vi "NewCore.vi"(8 "error in (no error)":errorcluster, 10 "ParamsArray":variant[](array[variant]), 11 "DoorNeedingSpell":refnum<class "DoorNeedingSpell.lvclass">) -> (0 "error out":errorcluster, 3 "DoorNeedingSpell":refnum<class "DoorNeedingSpell.lvclass">)   [LabVIEW 2020, in "DoorNeedingSpell.lvclass"]
uses:
  DoorNeedingSpell.lvclass
  Private/TypeDef/privateData.ctl
  DoorNeedingSpell.lvclass/DoorNeedingSpell.ctl
  Door/Door.lvclass
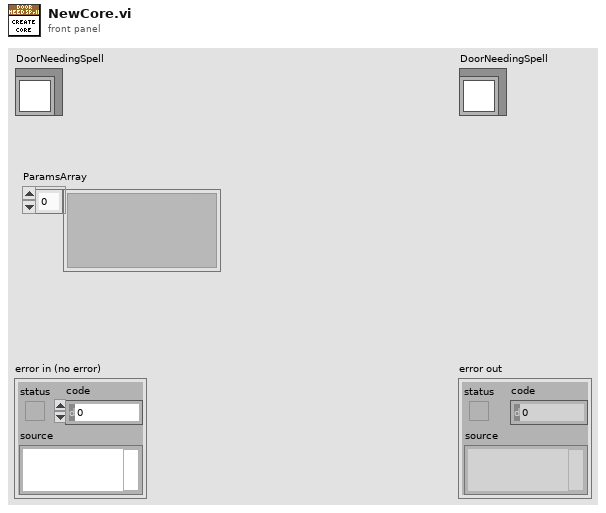
[diagram p1: front panel]
types:
  T1 = typedef "DoorNeedingSpell.lvclass/privateData.ctl" = cluster{"Dummy":i32}
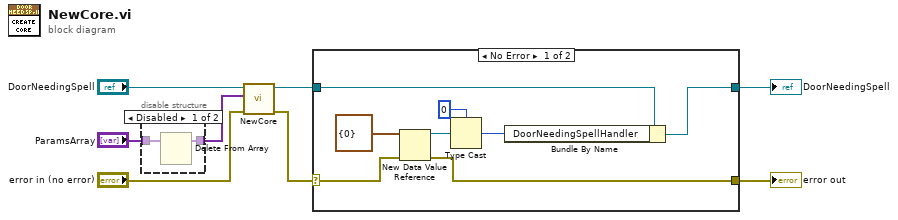
[diagram p0: block diagram]
diagram:
  n1 = disable-structure shown="Disabled" {
    disable-tunnel: "ParamsArray" -> [w10 w11]
    disable-tunnel: [w9 w11] -> w1
    frame Disabled {
      n2 = Delete From Array(array=w10) -> (array with subset deleted=w9:variant[])  [unwired: 2 in, 1 out]
    }
    frame Enabled {
    }
  }
  n3 = call-parent "NewCore.vi"("error in (no error)"="error in (no error)", "ParamsArray"=w1, "Door"="DoorNeedingSpell") -> ("error out"=w3:errorcluster, "Door"=w5:refnum<class "DoorNeedingSpell.lvclass">)  [unwired: 7 in]
  n4 = case shown="No Error" w3 {
    selector: w3 -> [w13 w21]
    tunnel: [w14 w21] -> w7
    tunnel: [w16 w20] -> w8
    tunnel: w5 -> [w15 w20]
    frame No Error {
      n5 = New Data Value Reference(data value=T1 {"Dummy"=0} ("privateData"), error in=w13) -> (data value reference=w19:refnum<data-value>, error out=w14:errorcluster)
      n6 = Type Cast(type=u32 0, x=w19) -> (*(type *) &x=w17:u32)
      n7 = Bundle By Name(cluster=w15, "DoorNeedingSpellHandler"=w17) -> (w16:refnum<class "DoorNeedingSpell.lvclass">)
    }
    frame Error {
    }
  }
  "error out" <- w7
  "DoorNeedingSpell" <- w8
